vi "Chassis Type Memory.vi"(7 "Operation":T1=enum."READ", 8 "Error In":errorcluster, 11 "Chassis type In":string) -> (0 "Error Out":errorcluster, 3 "Chassis type Out":string)   [LabVIEW 2011]
doc: "This VI will store Chassis type."
uses:
  Controls/INIT- READ - WRITE.ctl
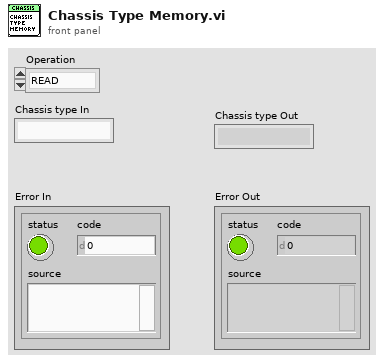
[diagram p1: front panel]
types:
  T1 = typedef "INIT- READ - WRITE.ctl" = enum16{"INIT", "READ", "WRITE"}
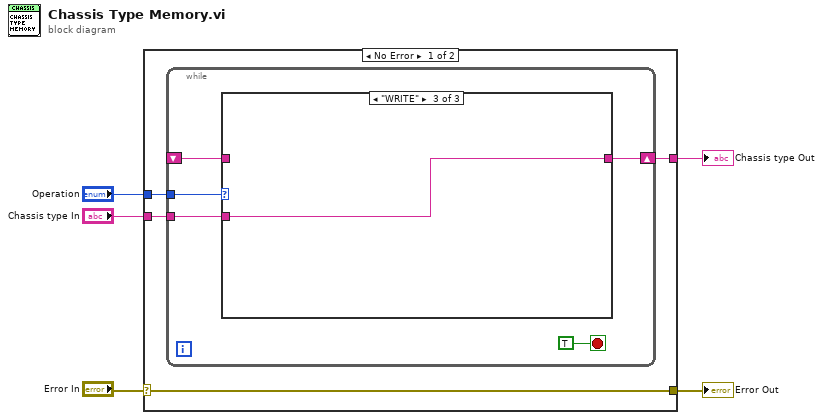
[diagram p0: block diagram]
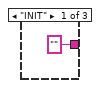
[diagram p2: hidden frame]
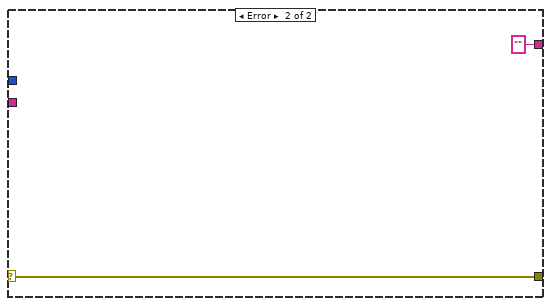
[diagram p4: hidden frame]
diagram:
  n1 = case shown="No Error" "Error In" {
    selector: "Error In" -> [w6 w19]
    tunnel: "Operation" -> [w9 _]
    tunnel: "Chassis type In" -> [w8 _]
    tunnel: [w7 "" ("Chassis type In")] -> w3
    tunnel: [w6 w19] -> w1
    frame No Error {
      n2 = while {
        tunnel: w9 -> [w14]
        tunnel: w8 -> [w13]
        shift-right: [w12] -> w7
        shift-left: _ -> [w11]
        stop <- TRUE stop-if-true
        n3 = case shown="\"WRITE\"" w14 {
          tunnel: w13 -> [_ _ w17]
          tunnel: ["" ("Chassis type") w16 w17] -> w12
          tunnel: w11 -> [_ w16 _]
          frame "INIT" {
          }
          frame "READ" {
          }
          frame "WRITE" {
          }
        }
      }
    }
    frame Error {
    }
  }
  "Chassis type Out" <- w3
  "Error Out" <- w1
